vi "FindWindow.vi"(3 "error in":errorcluster {"code" format="%.0x"}, 5 "Window Title":string) -> (0 "error out":errorcluster {"code" format="%.0x"}, 2 "HWND":u32 format="%x")   [LabVIEW 2012]
doc: "Retrieves a handle to the top-level window whose window name (titel) match the specified string. The VI does not perform a case-sensitive search."
uses:
  kernel32.dll
  user32.dll
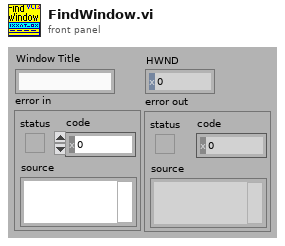
[diagram p1: front panel]
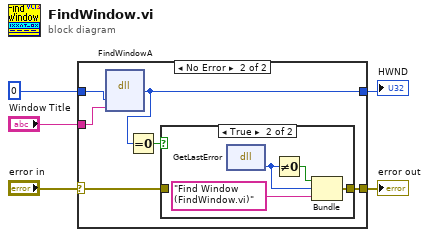
[diagram p0: block diagram]
diagram:
  n1 = case shown="No Error" "error in" {
    selector: "error in" -> [w7 w11]
    tunnel: [w7 w12] -> w4
    tunnel: [w6 w9] -> w3
    tunnel: "Window Title" -> [_ w10]
    tunnel: u32 0 ("MajorVersion") -> [w6 w8]
    frame Error {
    }
    frame No Error {
      n2 = dll-call lib="user32.dll" fn="FindWindowA"("pszClassName"=w8, "pszWindowName"=w10) -> (w9:u32)  [unwired: 5 in, 2 out]
      n3 = Equal To 0?(x=w9) -> (x = 0?=w13:bool)
      n4 = case shown="True" w13 {
        tunnel: [w14 w17] -> w12
        tunnel: w11 -> [w14 _]
        frame False {
        }
        frame True {
          n5 = dll-call lib="kernel32.dll" fn="GetLastError"() -> (w15:i32)  [unwired: 3 in, 2 out]
          n6 = Not Equal To 0?(x=w15) -> (x != 0?=w16:bool)
          n7 = Bundle(w16, w15, "Find Window (FindWindow.vi)") -> (w17:errorcluster)  [unwired: 1 in]
        }
      }
    }
  }
  "HWND" <- w3
  "error out" <- w4
